vi "Zone.vi"(8 "error in (no error)":errorcluster, 10 "Point":dbl[](array[numeric]), 11 "Zone in":refnum<class "Zone.lvclass">) -> (0 "error out":errorcluster, 2 "Zone":T1, 3 "Zone out":refnum<class "Zone.lvclass">)   [LabVIEW 2023, in "Zone.lvclass"]
uses:
  Zone.lvclass
  zones.ctl
  Zone.lvclass/Zone.ctl
  Field_class/Field.lvclass
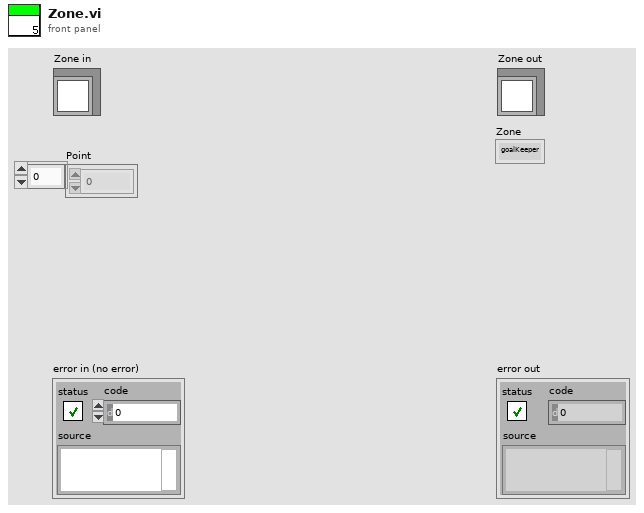
[diagram p1: front panel]
types:
  T1 = typedef "Zone.lvclass/zones.ctl" = enum16{"goalKeeper", "centerBack", "leftBack", "rightBack", "centerMidfield", "leftMidfield", "rightMidfield", "centerForward", "leftWing", "rightWing", "outsideField"}
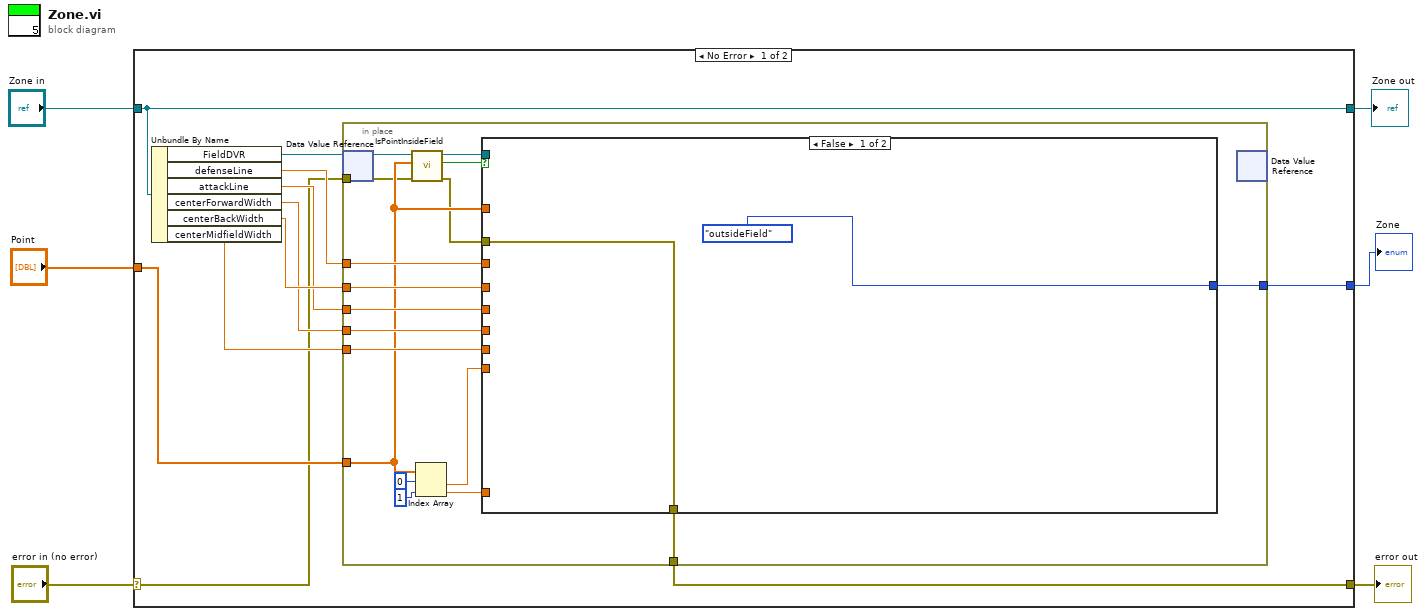
[diagram p0: block diagram]
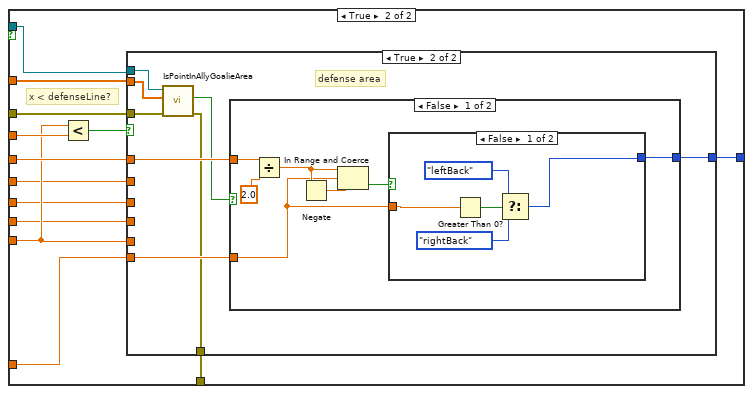
[diagram p2: hidden frame]
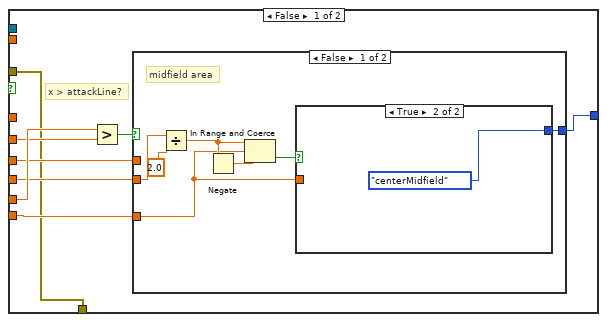
[diagram p3: hidden frame]
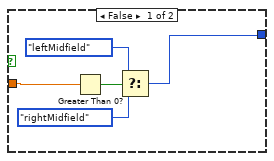
[diagram p4: hidden frame]
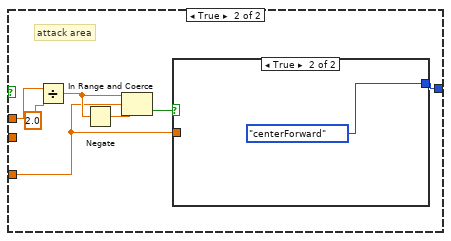
[diagram p5: hidden frame]
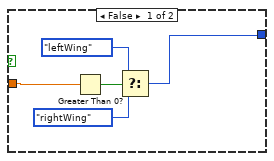
[diagram p6: hidden frame]
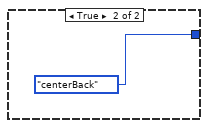
[diagram p7: hidden frame]
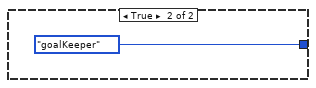
[diagram p8: hidden frame]
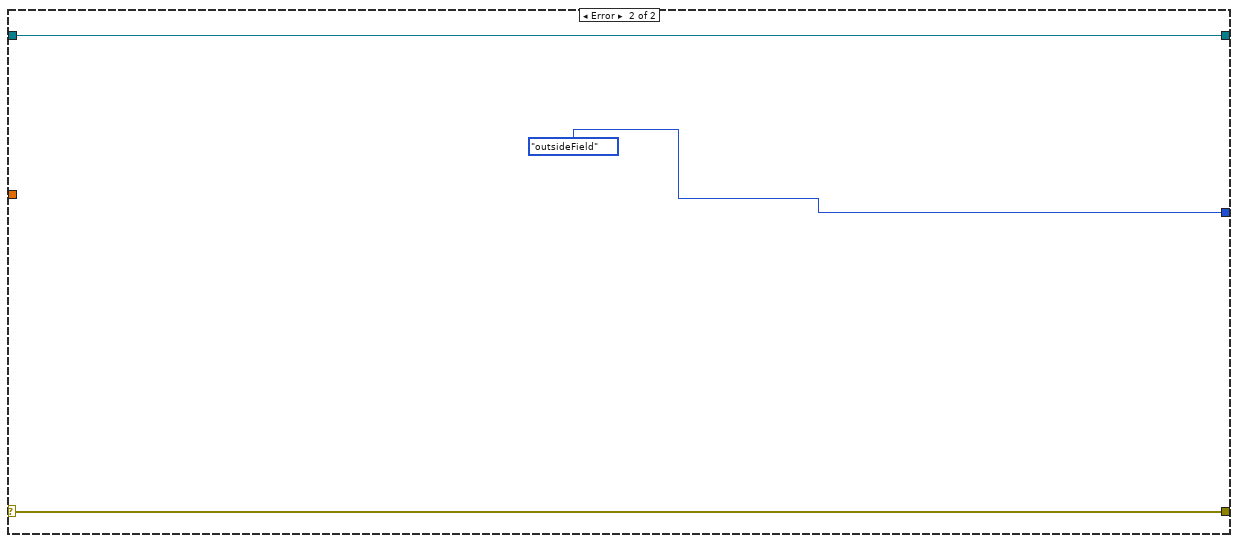
[diagram p9: hidden frame]
diagram:
  n1 = case shown="No Error" "error in (no error)" {
    selector: "error in (no error)" -> [w8 w108]
    tunnel: [w7 w108] -> w5
    tunnel: [w14 w107] -> w3
    tunnel: "Zone in" -> [w14 w107]
    tunnel: "Point" -> [w16 _]
    tunnel: [w15 zones."outsideField" ("Zone")] -> w1
    frame No Error {
      n2 = Unbundle By Name(w14) -> ("FieldDVR"=w17:refnum<data-value>, "defenseLine"=w13:dbl, "attackLine"=w11:dbl, "centerForwardWidth"=w10:dbl, "centerBackWidth"=w12:dbl, "centerMidfieldWidth"=w9:dbl)
      n3 = in-place {
        in-place-border: w16 -> [w21]
        in-place-border: [w32] -> w15
        in-place-border: w13 -> [w27]
        in-place-border: w12 -> [w26]
        in-place-border: w11 -> [w24]
        in-place-border: w10 -> [w23]
        in-place-border: w9 -> [w22]
        in-place-border: w8 -> [w20]
        in-place-border: [w18] -> w7
        n4 = in-place-dvr #1(w17) -> (w34:refnum<class "Field.lvclass">)  [unwired: 1 out]
        n5 = call-dynamic "IsPointInsideField.vi"("error in (no error)"=w20, "Point"=w21, "Field in"=w34) -> ("error out"=w19:errorcluster, "InsideField"=w33:bool, "Field out"=w31:refnum<class "Field.lvclass">)  [unwired: 6 in]
        n6 = Index Array(array=w21, index #1=0 ("index"), index #2=1 ("index")) -> (element #1=w28:dbl, element #2=w25:dbl)
        n7 = case shown="False" w33 {
          tunnel: [zones."outsideField" ("Zone") w48] -> w32
          tunnel: w31 -> [_ w40]
          tunnel: w28 -> [_ w44]
          tunnel: w27 -> [_ w46]
          tunnel: w26 -> [_ w47]
          tunnel: w25 -> [_ w45]
          tunnel: w24 -> [_ w43]
          tunnel: w23 -> [_ w42]
          tunnel: w22 -> [_ w41]
          tunnel: w21 -> [_ w39]
          tunnel: w19 -> [w35 w38]
          tunnel: [w35 w37] -> w18
          frame False {
          }
          frame True {
            # "x < defenseLine?"
            n8 = Less?(x=w44, y=w46) -> (x < y?=w49:bool)
            n9 = case shown="True" w49 {
              tunnel: [w51 w90] -> w48
              tunnel: w47 -> [_ w91]
              tunnel: w45 -> [w54 w89]
              tunnel: w44 -> [w56 _]
              tunnel: w43 -> [w55 _]
              tunnel: w42 -> [w53 _]
              tunnel: w41 -> [w52 _]
              tunnel: w40 -> [_ w88]
              tunnel: w39 -> [_ w87]
              tunnel: w38 -> [w50 w85]
              tunnel: [w50 w84] -> w37
              frame False {
                # "x > attackLine?"
                n10 = Greater?(x=w56, y=w55) -> (0:w57:bool)
                n11 = case shown="False" w57 {
                  tunnel: w54 -> [w59 w73]
                  tunnel: w53 -> [_ w72]
                  tunnel: w52 -> [w60 _]
                  tunnel: [w58 w71] -> w51
                  frame False {
                    # "midfield area"
                    n12 = Divide(x=w60, y=2.0) -> (x/y=w62:dbl)
                    n13 = Negate(x=w62) -> (-x=w63:dbl)
                    n14 = In Range and Coerce(upper limit=w62, x=w59, lower limit=w63) -> (In Range?=w61:bool)  [unwired: 1 out]
                    n15 = case shown="True" w61 {
                      tunnel: [w66 zones."centerMidfield" ("Zone")] -> w58
                      tunnel: w59 -> [w68 _]
                      frame False {
                        n16 = Greater Than 0?(x=w68) -> (x > 0?=w69:bool)
                        n17 = Select(t=zones."leftMidfield" ("Zone"), s=w69, f=zones."rightMidfield") -> (s? t:f=w66:T1)
                      }
                      frame True {
                      }
                    }
                  }
                  frame True {
                    # "attack area"
                    n18 = Divide(x=w72, y=2.0) -> (x/y=w75:dbl)
                    n19 = Negate(x=w75) -> (-x=w76:dbl)
                    n20 = In Range and Coerce(upper limit=w75, x=w73, lower limit=w76) -> (In Range?=w74:bool)  [unwired: 1 out]
                    n21 = case shown="True" w74 {
                      tunnel: [w79 zones."centerForward" ("Zone")] -> w71
                      tunnel: w73 -> [w81 _]
                      frame False {
                        n22 = Greater Than 0?(x=w81) -> (x > 0?=w82:bool)
                        n23 = Select(t=zones."leftWing" ("Zone"), s=w82, f=zones."rightWing") -> (s? t:f=w79:T1)
                      }
                      frame True {
                      }
                    }
                  }
                }
              }
              frame True {
                # "defense area"
                n24 = call-dynamic "IsPointInAllyGoalieArea.vi"("error in (no error)"=w85, "Point"=w87, "Field in"=w88) -> ("error out"=w84:errorcluster, "InGoalieArea"=w86:bool)  [unwired: 6 in, 1 out]
                n25 = case shown="False" w86 {
                  tunnel: w91 -> [w97 _]
                  tunnel: [w93 zones."goalKeeper" ("Zone")] -> w90
                  tunnel: w89 -> [w92 _]
                  frame False {
                    n26 = Divide(x=w97, y=2.0) -> (x/y=w95:dbl)
                    n27 = Negate(x=w95) -> (-x=w96:dbl)
                    n28 = In Range and Coerce(upper limit=w95, x=w92, lower limit=w96) -> (In Range?=w94:bool)  [unwired: 1 out]
                    n29 = case shown="False" w94 {
                      tunnel: [w100 zones."centerBack" ("Zone")] -> w93
                      tunnel: w92 -> [w102 _]
                      frame False {
                        n30 = Greater Than 0?(x=w102) -> (x > 0?=w103:bool)
                        n31 = Select(t=zones."leftBack" ("Zone"), s=w103, f=zones."rightBack") -> (s? t:f=w100:T1)
                      }
                      frame True {
                      }
                    }
                  }
                  frame True {
                  }
                }
              }
            }
          }
        }
        n32 = in-place-dvr #1() -> ()  [unwired: 1 in, 2 out]
      }
    }
    frame Error {
    }
  }
  "error out" <- w5
  "Zone out" <- w3
  "Zone" <- w1
